vi "Start Rx.vi"(8 "error in (no error)":errorcluster, 11 "Cluster":T1) -> (0 "error out":errorcluster)   [LabVIEW 2015, in "QCA_DUT_Func.lvlib"]
doc: "DLL_QMSL_AEROFLEX void _stdcall StartRx(unsigned int channel,unsigned int channel2,unsigned int rxMode,unsigned int rxChain,unsigned int wlanMode,unsigned int rateMask,unsigned int antenna ,unsigned int bandwidth );"
uses:
  QCA_DUT_Func.lvlib
  QCA_DUT_Func.dll
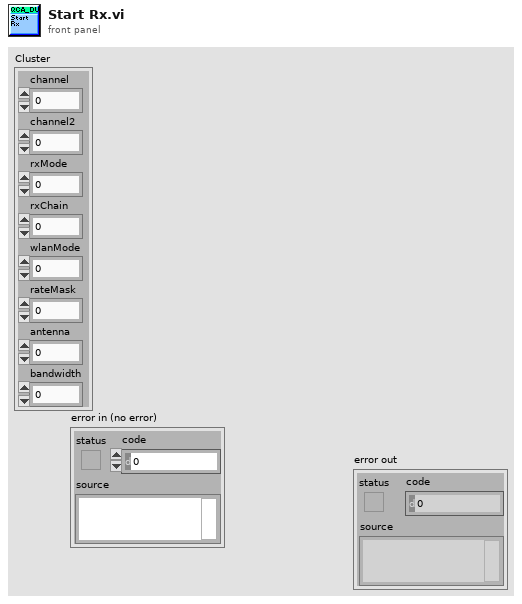
[diagram p1: front panel]
types:
  T1 = cluster{"channel":u32, "channel2":u32, "rxMode":u32, "rxChain":u32, "wlanMode":u32, "rateMask":u32, "antenna":u32, "bandwidth":u32}
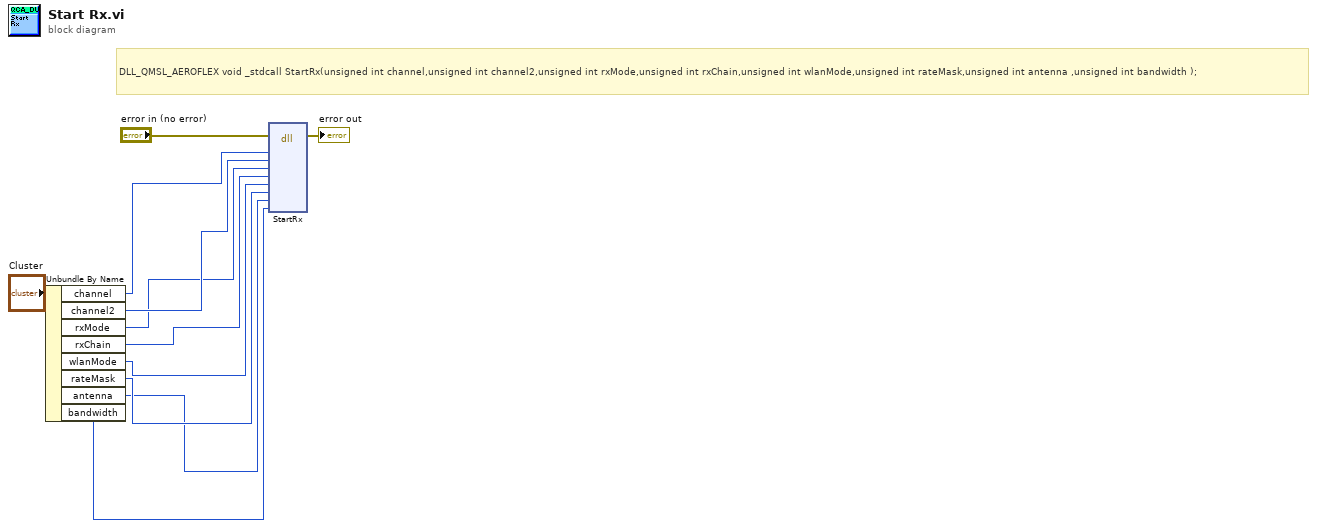
[diagram p0: block diagram]
diagram:
  # "DLL_QMSL_AEROFLEX void _stdcall StartRx(unsigned int channel,unsigned int channel2,unsigned int rxMode,unsigned int rxChain,unsigned int wlanMode,unsigned int rateMask,unsigned int antenna ,unsigned int bandwidth );"
  n1 = Unbundle By Name("Cluster") -> ("channel"=w8:u32, "channel2"=w7:u32, "rxMode"=w6:u32, "rxChain"=w5:u32, "wlanMode"=w4:u32, "rateMask"=w3:u32, "antenna"=w2:u32, "bandwidth"=w1:u32)
  n2 = dll-call lib="D:/4-Up-WLAN-Test-System/DUT Control/DUT/dut_control/QCA_DUT_Func.dll" fn="StartRx"(error in="error in (no error)", "channel"=w8, "channel2"=w7, "rxMode"=w6, "rxChain"=w5, "wlanMode"=w4, "rateMask"=w3, "antenna"=w2, "bandwidth"=w1) -> (error out=→"error out":errorcluster)  [unwired: 11 in, 1 out]
